vi "Create Request-JSONtext.vi"(6 "notification?":bool, 8 "error in (no error)":errorcluster, 9 "params":variant, 10 "method":string) -> (0 "error out":errorcluster, 2 "<JSON>":string, 4 "id":string)   [LabVIEW 2019, in "JSON-RPC.lvclass"]
uses:
  JSON-RPC.lvclass
  <vilib>/Utility/MD5Checksum.llb/MD5Checksum string.vi
  <vilib>/JDP Science/JSONtext/support/Format JSON Object.vi
  6eedbf92-275d-42c0-90bb-b913601e88e9.vi
  <vilib>/Utility/Data Type/NI_Data Type.lvlib
  <vilib>/JDP Science/JSONtext/JSONtext.lvlib
  6cd1d572-2af6-48e8-9b38-c51782860e23.vi
  7c5521bf-cb07-444f-843e-f9f289aa2aae.vi
  f6ae5555-b15c-4e52-b9b9-d6341c380ca9.vi
  typedefs/Request--Cluster.ctl
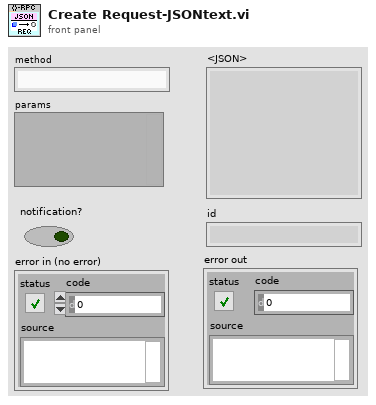
[diagram p1: front panel]
types:
  T1 = typedef "NI_Data Type.lvlib/Data Type.ctl" = enum8{"Invalid Type", "Void", "I8", "I16", "I32", "I64", "U8", "U16", "U32", "U64", "Single Float", "Double Float", "Extended Float", "Single Complex", "Double Complex", "Extended Complex", "Enum U8", "Enum U16", "Enum U32", "Enum U64", "Single Float With Unit", "Double Float With Unit", "Extended Float With Unit", "Single Complex with Unit", "Double Complex with Unit", "Extended Complex with Unit", "Boolean", "String", "Path", "Picture", "Tag", "Array", "Cluster", "Variant", "LV Variant", "Waveform", "Timestamp", "Digital Waveform", "Digital Data", "ExpressData", "Refnum", "External Data", "VI", "Poly VI", "LabVIEW Class Instance", "Fixed Point", "Set Collection", "Map Collection"}
  T2 = typedef "JSON-RPC.lvclass/Request--Cluster.ctl" = cluster{"jsonrpc":string, "method":string, "params":string, "id":string}
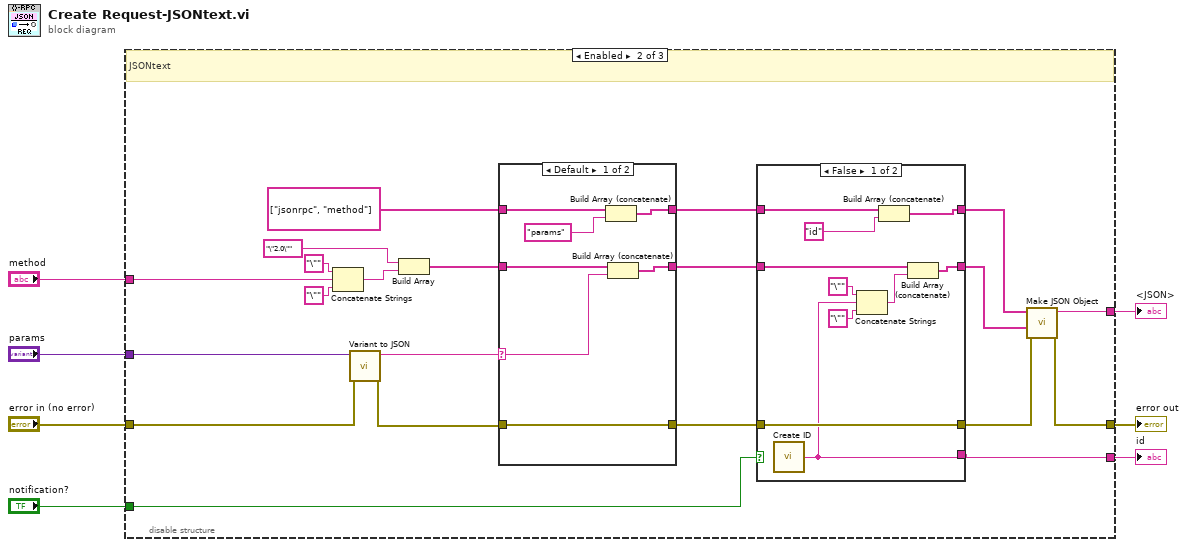
[diagram p0: block diagram]
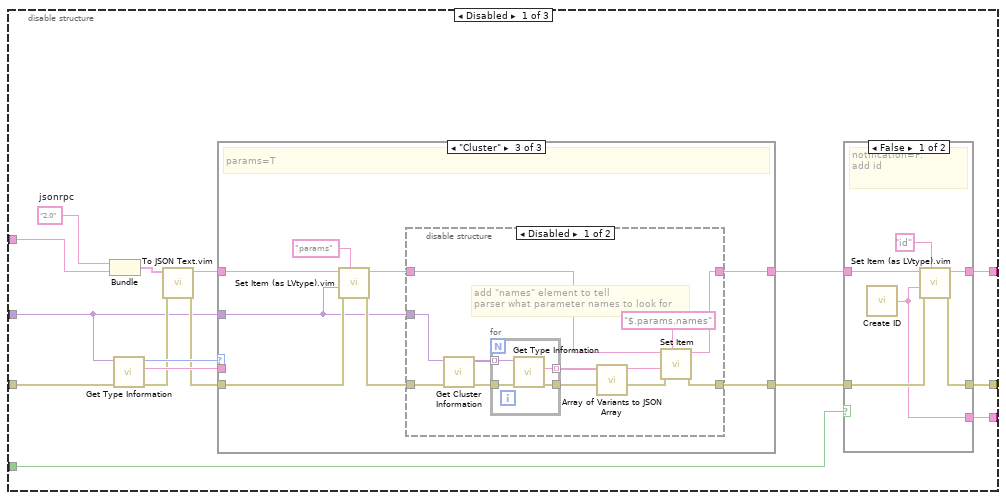
[diagram p2: hidden frame]
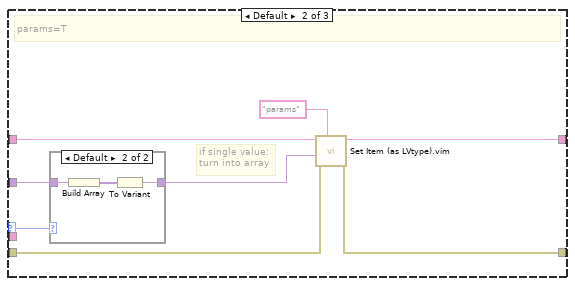
[diagram p4: hidden frame]
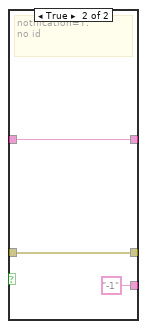
[diagram p7: hidden frame]
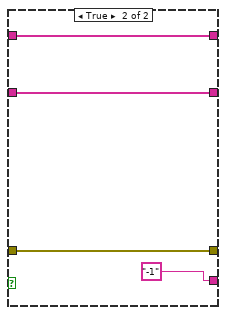
[diagram p8: hidden frame]
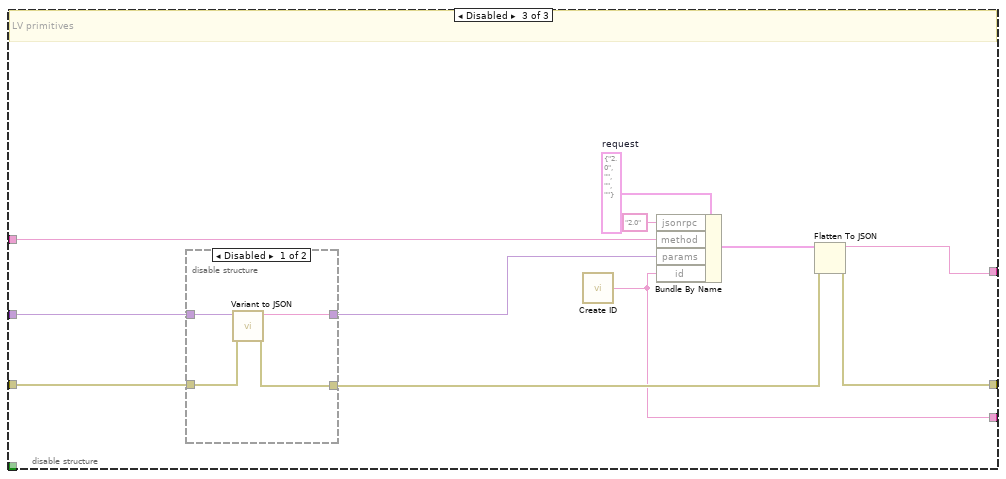
[diagram p10: hidden frame]
diagram:
  n1 = disable-structure shown="Enabled" {
    disable-tunnel: "error in (no error)" -> [w23 w80 w128]
    disable-tunnel: [w22 w93 w122] -> w6
    disable-tunnel: [w21 w92 w121] -> w5
    disable-tunnel: "notification?" -> [w20 w88 _]
    disable-tunnel: [w16 w82 w118] -> w3
    disable-tunnel: "method" -> [w12 w77 w125]
    disable-tunnel: "params" -> [w8 w81 w126]
    frame Disabled {
      w13 = "2.0"  # jsonrpc
      n2 = Bundle("jsonrpc"=w13, "method"=w12) -> (w14:cluster{"jsonrpc":string, "method":string})  [unwired: 1 in]
      n3 = call <vilib>:"Get Type Information.vi"("error in (no error)"=w23, "variant"=w8) -> ("error out"=w11:errorcluster, "name"=w15:string, "type"=w19:T1)  [unwired: 5 in, 2 out]
      n4 = call "To JSON Text.vim"("error in (no error)"=w11, "Anything"=w14) -> ("error out"=w10:errorcluster, "<JSON>"=w9:string)  [unwired: 8 in]
      n5 = case shown="\"Cluster\"" w19 {
        selector: w19 -> [_ w32 _]
        tunnel: [w25 w28 w45] -> w17
        tunnel: [w24 w27 w44] -> w18
        tunnel: w10 -> [w25 w26 w41]
        tunnel: w9 -> [w24 w33 w42]
        tunnel: w8 -> [_ w31 w38]
        tunnel: w15 -> [_ _ _]
        frame "Void" {
          # "no params"
        }
        frame Default {
          # "if single value:\nturn into array"
          # "params=T"
          n6 = case shown="Default" w32 {
            tunnel: w31 -> [w34 w37]
            tunnel: [w34 w36] -> w29
            frame "Array" {
            }
            frame Default {
              n7 = Build Array(w37) -> (w35:variant[])
              n8 = To Variant(anything=w35) -> (Variant=w36:variant)
            }
          }
          n9 = call "Set Item (as LVtype).vim"("$Path or Item Name"="params" ("Object (or Item) Path"), "error in (no error)"=w26, "Anything"=w29, "JSON"=w33) -> ("error out"=w28:errorcluster, "<JSON>"=w27:string)  [unwired: 4 in, 1 out]
        }
        frame "Cluster" {
          # "params=T"
          n10 = call "Set Item (as LVtype).vim"("$Path or Item Name"="params" ("Object (or Item) Path"), "error in (no error)"=w41, "Anything"=w38, "JSON"=w42) -> ("error out"=w40:errorcluster, "<JSON>"=w39:string)  [unwired: 4 in, 1 out]
          n11 = disable-structure shown="Disabled" {
            disable-tunnel: [w54 w62] -> w45
            disable-tunnel: w38 -> [w50 _]
            disable-tunnel: w40 -> [w49 w62]
            disable-tunnel: w39 -> [w48 w63]
            disable-tunnel: [w46 w63] -> w44
            frame Disabled {
              # "add \"names\" element to tell\nparser what parameter names to look for"
              n12 = call <vilib>:"Get Cluster Information.vi"("error in (no error)"=w49, "variant"=w50) -> ("error out"=w57:errorcluster, "cluster elements"=w56:variant[])  [unwired: 8 in]
              n13 = for {
                tunnel: w56 -> [w61] mode=indexing
                tunnel: [w60] -> w51 mode=indexing
                tunnel: w57 -> [w59]
                tunnel: [w58] -> w47
                n14 = call <vilib>:"Get Type Information.vi"("error in (no error)"=w59, "variant"=w61) -> ("error out"=w58:errorcluster, "name"=w60:string)  [unwired: 5 in, 3 out]
              }
              n15 = call <vilib>:"Array of Variants to JSON Array.vi"("error in (no error)"=w47, "Array of Variants"=w51) -> ("error out"=w52:errorcluster, "<JSON>"=w53:string)  [unwired: 8 in]
              n16 = call <vilib>:"Set Item.vi"("$Path or Item Name"="$.params.names", "error in (no error)"=w52, "JSON to Insert"=w53, "JSON"=w48) -> ("error out"=w54:errorcluster, "<JSON>"=w46:string)  [unwired: 4 in, 1 out]
            }
            frame Enabled {
            }
          }
        }
      }
      n17 = case shown="False" w20 {
        tunnel: w18 -> [w69 w72]
        tunnel: [w68 w72] -> w22
        tunnel: w17 -> [w66 w71]
        tunnel: [w67 w71] -> w21
        tunnel: [w64 "-1" ("id")] -> w16
        frame False {
          # "notification=F:\nadd id"
          n18 = call "Create ID.vi"() -> ("id"=w64:string)
          n19 = call "Set Item (as LVtype).vim"("$Path or Item Name"="id", "error in (no error)"=w66, "Anything"=w64, "JSON"=w69) -> ("error out"=w67:errorcluster, "<JSON>"=w68:string)  [unwired: 4 in, 1 out]
        }
        frame True {
          # "notification=T:\nno id"
        }
      }
    }
    frame Enabled {
      # "JSONtext"
      n20 = Concatenate Strings("\"" ("string"), w77, "\"" ("string")) -> (w74:string)
      n21 = call "Variant to JSON.vi"("error in (no error)"=w80, "variant"=w81) -> ("error out"=w79:errorcluster, "<JSON>"=w78:string)  [unwired: 8 in]
      n22 = Build Array("\"2.0\"", w74) -> (w91:string[])
      n23 = case shown="Default" w78 {
        selector: w78 -> [w108 _]
        tunnel: [w109 w117] -> w87
        tunnel: w91 -> [w111 w117]
        tunnel: string[] ["jsonrpc", "method"] -> [w114 w116]
        tunnel: [w112 w116] -> w89
        tunnel: w79 -> [w110 w115]
        tunnel: [w110 w115] -> w83
        frame Default {
          n24 = Build Array (concatenate)(w114, "params" ("String")) -> (w112:string[])
          n25 = Build Array (concatenate)(w111, w108) -> (w109:string[])
        }
        frame "null" {
        }
      }
      n26 = case shown="False" w88 {
        tunnel: w89 -> [w101 w106]
        tunnel: w87 -> [w99 w107]
        tunnel: [w102 w107] -> w86
        tunnel: [w100 w106] -> w85
        tunnel: [w98 w105] -> w84
        tunnel: w83 -> [w98 w105]
        tunnel: [w94 "-1" ("id")] -> w82
        frame False {
          n27 = call "Create ID.vi"() -> ("id"=w94:string)
          n28 = Concatenate Strings("\"" ("string"), w94, "\"" ("string")) -> (w95:string)
          n29 = Build Array (concatenate)(w101, "id" ("String")) -> (w100:string[])
          n30 = Build Array (concatenate)(w99, w95) -> (w102:string[])
        }
        frame True {
        }
      }
      n31 = call <vilib>:"Make JSON Object.vi"("error in (no error)"=w84, "JSON Items"=w86, "Item Names"=w85) -> ("error out"=w92:errorcluster, "<JSON>"=w93:string)  [unwired: 7 in]
    }
    frame Disabled {
      w127 = T2 {"jsonrpc"="2.0", "method"="", "params"="", "id"=""}  # request
      # "LV primitives"
      n32 = disable-structure shown="Disabled" {
        disable-tunnel: w128 -> [w132 w134]
        disable-tunnel: w126 -> [w131 w133]
        disable-tunnel: [w130 w134] -> w120
        disable-tunnel: [w129 w133] -> w119
        frame Disabled {
          n33 = call "Variant to JSON.vi"("error in (no error)"=w132, "variant"=w131) -> ("error out"=w130:errorcluster, "<JSON>"=w129:string)  [unwired: 8 in]
        }
        frame Enabled {
        }
      }
      n34 = call "Create ID.vi"() -> ("id"=w118:string)
      n35 = Bundle By Name(cluster=w127, "jsonrpc"="2.0", "method"=w125, "params"=w119, "id"=w118) -> (w123:T2)
      n36 = Flatten To JSON(anything=w123, error in (no error)=w120) -> (JSON string=w122:string, 11:w121:errorcluster)  [unwired: 1 in]
    }
  }
  "error out" <- w5
  "<JSON>" <- w6
  "id" <- w3
